vi "Create RX and TX FIFOs.vi"(8 "error in":errorcluster, 10 "Values for Naming":T1={"Bus Number"=1, "Device Number"=1, "Channel Number"=1} {"Channel Number" min=0 step=1; "Device Number" min=0 step=1; "Bus Number" min=0 step=1}, 11 "New Virtual Folder":refnum<vi>) -> (0 "error out":errorcluster, 3 "Comm FIFOs Virtual Folder":refnum<vi>)   [LabVIEW 2014, in "SPI Engine Scripting.lvlib"]
doc: "Calls VIs to name and create RX and TX FIFOs."
uses:
  SPI Engine Scripting.lvlib
  State Machine/Controls/Values for Naming.ctl
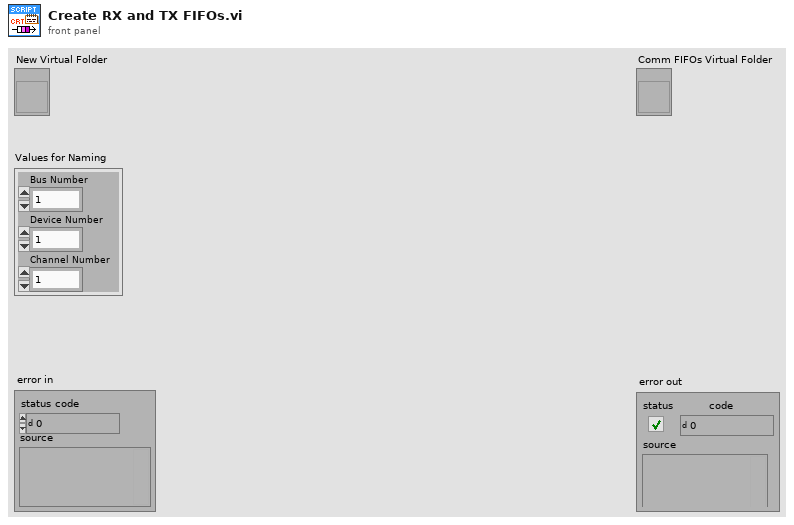
[diagram p1: front panel]
types:
  T1 = typedef "SPI Engine Scripting.lvlib/Values for Naming.ctl" = cluster{"Bus Number":i32, "Device Number":i32, "Channel Number":i32}
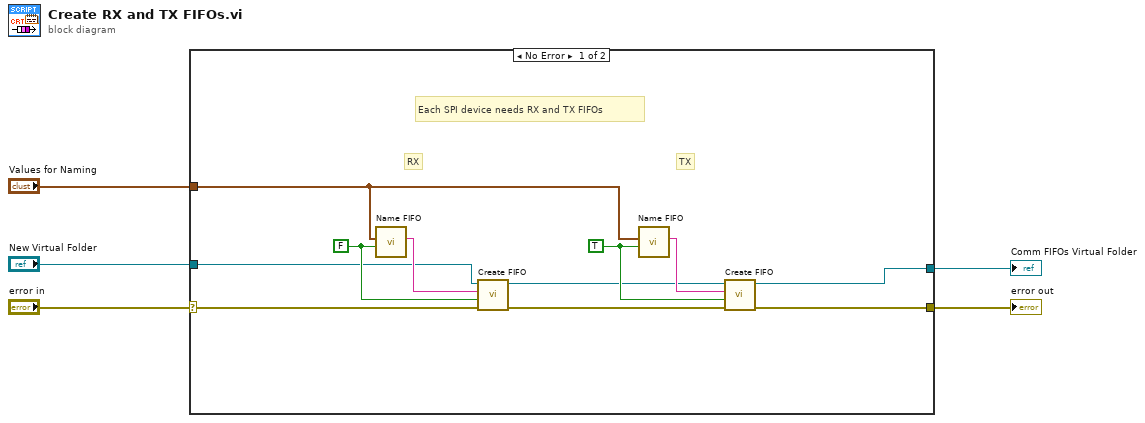
[diagram p0: block diagram]
diagram:
  n1 = case shown="No Error" "error in" {
    selector: "error in" -> [w14 w18]
    tunnel: [w15 w18] -> w4
    tunnel: "New Virtual Folder" -> [w7 w17]
    tunnel: [w16 w17] -> w2
    tunnel: "Values for Naming" -> [w13 _]
    frame No Error {
      w8 = TRUE
      w9 = FALSE
      # "TX"
      # "RX"
      # "Each SPI device needs RX and TX FIFOs"
      n2 = call "Name FIFO.vi"("TX?"=w9, "Values for Naming"=w13) -> ("FIFO Name"=w12:string)  [unwired: 9 in]
      n3 = call "Create FIFO.vi"("error in (no error)"=w14, "TX?"=w9, "FIFO Name"=w12, "Comm FIFOs Virtual Folder"=w7) -> ("error out"=w10:errorcluster, "Comm FIFOs Virtual Folder"=w6:refnum<vi>)  [unwired: 6 in]
      n4 = call "Name FIFO.vi"("TX?"=w8, "Values for Naming"=w13) -> ("FIFO Name"=w11:string)  [unwired: 9 in]
      n5 = call "Create FIFO.vi"("error in (no error)"=w10, "TX?"=w8, "FIFO Name"=w11, "Comm FIFOs Virtual Folder"=w6) -> ("error out"=w15:errorcluster, "Comm FIFOs Virtual Folder"=w16:refnum<vi>)  [unwired: 6 in]
    }
    frame Error {
    }
  }
  "error out" <- w4
  "Comm FIFOs Virtual Folder" <- w2
